vi "Read Gui_MainCtrl.vi"(8 "error in (no error)":errorcluster, 11 "GUI_Handler_Main in":refnum<class "GUI_Handler_Main.lvclass">) -> (0 "error out":errorcluster, 2 "Gui_MainCtrl":T1, 3 "GUI_Handler_Main out":refnum<class "GUI_Handler_Main.lvclass">)   [LabVIEW 2019, in "GUI_Handler_Main.lvclass"]
uses:
  GUI_Handler_Main.lvclass
  GUI_Handler_Main.lvclass/GUI_Handler_Main.ctl
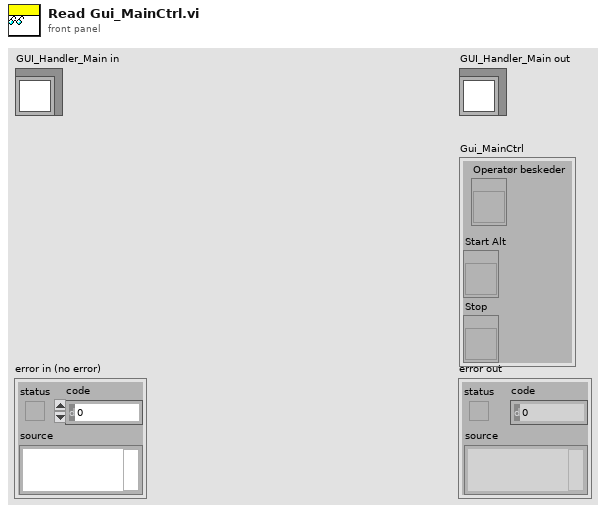
[diagram p1: front panel]
types:
  T1 = cluster{"Start Alt":refnum<vi>, "Stop":refnum<vi>, "Operatør beskeder":refnum<vi>}
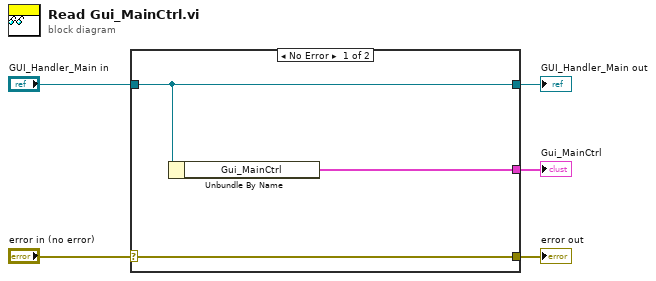
[diagram p0: block diagram]
diagram:
  n1 = case shown="No Error" "error in (no error)" {
    selector: "error in (no error)" -> [w8 w9]
    tunnel: [w8 w9] -> w4
    tunnel: [w7 w10] -> w2
    tunnel: "GUI_Handler_Main in" -> [w7 w10]
    tunnel: [w6 _] -> w1
    frame No Error {
      n2 = Unbundle By Name(w7) -> ("Gui_MainCtrl"=w6:T1)
    }
    frame Error {
    }
  }
  "error out" <- w4
  "GUI_Handler_Main out" <- w2
  "Gui_MainCtrl" <- w1
